vi "Read Async Elements.vi"(11 "Base Async Elements in":refnum<class "Base Async Elements.lvclass">) -> (2 "Async Elements":refnum<queue>)   [LabVIEW 2020, in "jettl.lvlib" / "Base Async Elements.lvlib" / "Base Async Elements.lvclass"]
uses:
  Base Async Elements.lvclass
  Attributes/Attributes.lvclass
  Base Async Elements.lvclass/Base Async Elements.ctl
  Async Elements.ctl
  jettl.lvlib
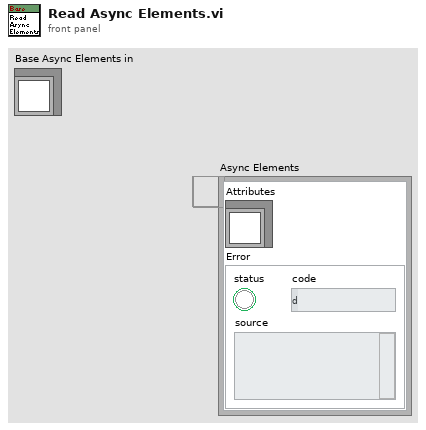
[diagram p1: front panel]
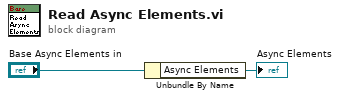
[diagram p0: block diagram]
diagram:
  n1 = Unbundle By Name("Base Async Elements in") -> ("Async Elements"=→"Async Elements":refnum<queue>)
